vi "peakFinding getPeakIdx.vi"(5 "window":i32=5, 7 "dt":dbl=1.0 format="%#_13g", 9 "ampTh":dbl=-inf, 10 "slopeTh":dbl=-inf, 11 "yData":dbl[](array[numeric])) -> (1 "rightIdx":i32[](array[numeric]), 2 "leftIdx":i32[](array[numeric]), 3 "peakIdx":i32[](array[numeric]))   [LabVIEW 2018]
uses:
  <vilib>/Analysis/5stat.llb/RMS (DBL).vi
  <vilib>/ptbypt/NI_PtbyPt.lvlib
  <vilib>/Analysis/NI_AALPro.lvlib
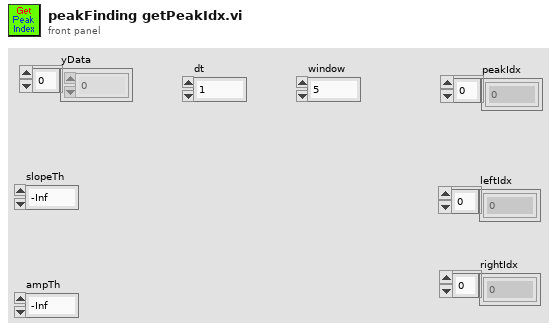
[diagram p1: front panel]
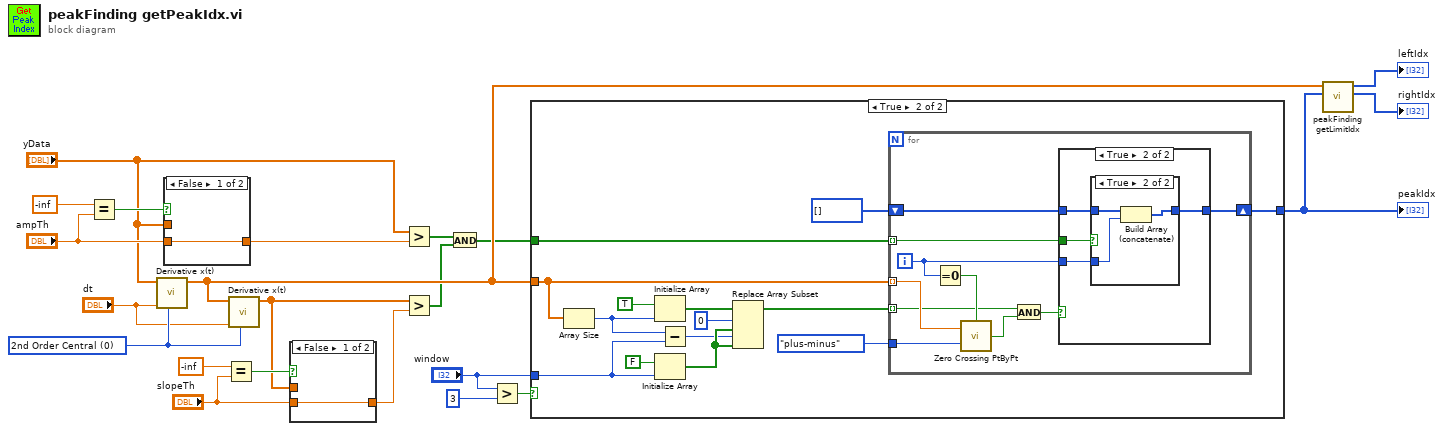
[diagram p0: block diagram]
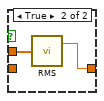
[diagram p6: hidden frame]
diagram:
  w21 = u16 0 items=["2nd Order Central", "4th Order Central", "Forward", "Backward"] ("method")
  n1 = Equal?(x=-inf ("y"), y="ampTh") -> (x = y?=w22:bool)
  n2 = call <vilib>:"Derivative x(t).vi"("method"=w21, "dt"="dt", "X"="yData") -> ("dX/dt"=w10:dbl[])  [unwired: 7 in, 1 out]
  n3 = case shown="False" w22 {
    tunnel: "yData" -> [_ w25]
    tunnel: "ampTh" -> [w23 _]
    tunnel: [w23 w24] -> w4
    frame False {
    }
    frame True {
      n4 = call-poly <vilib>:"RMS.vi"("X"=w25) -> ("rms value"=w24:dbl)  [unwired: 1 out]
    }
  }
  n5 = Equal?(x=-inf ("y"), y="slopeTh") -> (x = y?=w19:bool)
  n6 = call <vilib>:"Derivative x(t).vi"("method"=w21, "dt"="dt", "X"=w10) -> ("dX/dt"=w7:dbl[])  [unwired: 7 in, 1 out]
  n7 = case shown="False" w19 {
    tunnel: w7 -> [_ _]
    tunnel: [w26 w27] -> w6
    tunnel: "slopeTh" -> [w26 w27]
    frame False {
    }
    frame True {
    }
  }
  n8 = Greater?(x="yData", y=w4) -> (0:w2:bool[])
  n9 = Greater?(x=w7, y=w6) -> (0:w3:bool[])
  n10 = And(x=w2, y=w3) -> (x .and. y?=w1:bool[])
  n11 = Greater?(x="window", y=3) -> (0:w14:bool)
  n12 = case shown="True" w14 {
    tunnel: "window" -> [_ w32]
    tunnel: w10 -> [_ w29]
    tunnel: [_ w39] -> w13
    tunnel: w1 -> [_ w28]
    frame False {
    }
    frame True {
      n13 = Array Size(array=w29) -> (size(s)=w33:i32)
      n14 = Initialize Array(TRUE, w33) -> (w36:bool[])
      n15 = Initialize Array(FALSE, w32) -> (w34:bool[])
      n16 = Subtract(x=w33, y=w32) -> (x-y=w31:i32)
      n17 = Replace Array Subset(array=w36, new element #1=w34, index #1=0 ("index"), new element #2=w34, index #2=w31) -> (w30:bool[])
      n18 = for {
        shift-right: [w50] -> w39
        shift-left: i32[] [] -> [w51]
        tunnel: enum16{"either", "minus-plus", "plus-minus"}."plus-minus" ("direction") -> [w49]
        tunnel: w30 -> [w44] mode=indexing
        tunnel: w29 -> [w45] mode=indexing
        tunnel: w28 -> [w42] mode=indexing
        i -> [w47]
        n19 = Equal To 0?(x=w47) -> (x = 0?=w48:bool)
        n20 = call <vilib>:"Zero Crossing PtByPt.vi"("initialize"=w48, "direction"=w49, "input data point"=w45) -> ("crossing"=w43:bool)
        n21 = And(x=w44, y=w43) -> (x .and. y?=w46:bool)
        n22 = case shown="True" w46 {
          tunnel: w51 -> [w52 w56]
          tunnel: w47 -> [_ w55]
          tunnel: [w52 w54] -> w50
          tunnel: w42 -> [_ w53]
          frame False {
          }
          frame True {
            n23 = case shown="True" w53 {
              tunnel: w56 -> [w57 w60]
              tunnel: w55 -> [_ w59]
              tunnel: [w57 w58] -> w54
              frame False {
              }
              frame True {
                n24 = Build Array (concatenate)(w60, w59) -> (w58:i32[])
              }
            }
          }
        }
      }
    }
  }
  "peakIdx" <- w13
  n25 = call "peakFinding getLimitIdx.vi"("peakIdxArray"=w13, "1stDiffData"=w10) -> ("rightIdx"=→"rightIdx":i32[], "leftIdx"=→"leftIdx":i32[])  [unwired: 7 in, 1 out]
